vi "Read G08 Specific.vi"(8 "error in (no error)":errorcluster, 11 "BME_DG_G08_Chnl in":refnum<class "BME_DG_G08_Chnl.lvclass">) -> (0 "error out":errorcluster, 1 "Output Offset":u32, 2 "Pulse Width (µs)":dbl=0.005 min=0.0 max=8947840.0 format="%.6f", 3 "BME_DG_G08_Chnl out":refnum<class "BME_DG_G08_Chnl.lvclass">)   [LabVIEW 2009, in "POLARIS BME DG.lvlib" / "BME_DG_G08_Chnl.lvclass"]
uses:
  BME_DG_G08_Chnl.lvclass
  BME_DG_G08_Chnl.lvclass/BME_DG_G08_Chnl.ctl
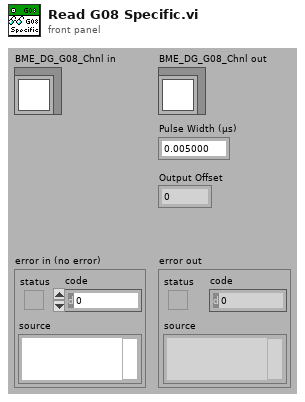
[diagram p1: front panel]
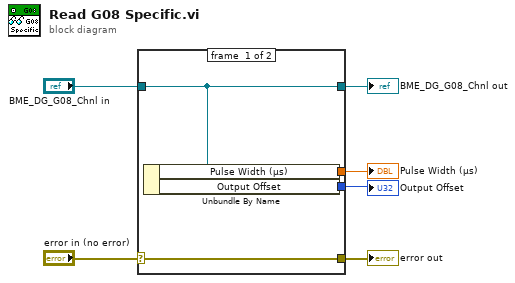
[diagram p0: block diagram]
diagram:
  n1 = case shown="No Error" "error in (no error)" {
    selector: "error in (no error)" -> [w10 w11]
    tunnel: [w10 w11] -> w5
    tunnel: [w9 w12] -> w3
    tunnel: "BME_DG_G08_Chnl in" -> [w9 w12]
    tunnel: [w8 _] -> w2
    tunnel: [w7 _] -> w1
    frame #0 {
      n2 = Unbundle By Name(w9) -> ("Pulse Width (µs)"=w8:dbl, "Output Offset"=w7:u32)
    }
    frame #1 {
    }
  }
  "error out" <- w5
  "BME_DG_G08_Chnl out" <- w3
  "Pulse Width (µs)" <- w2
  "Output Offset" <- w1
